vi "Start Stream.vi"(8 "error in (no error)":errorcluster, 10 "Camera Settings":T1={"Exposure Time (ms)"=100.0, "Binning"=enum."2x2", "Scan Mode"=0, "Frames to Acquire"=1000.0, "Pixel Correction"=FALSE, "Frames to Skip"=0, "File Path"=path "", "Duty cycle"=0.0, "ALEX"=FALSE, "Shutter Enable"=[], "fluidics trigger, ms (0=disabled)"=0.0, "Bit Depth"=0, "Image Width (px)"=0, "Image Height (px)"=0, "Horizontal Offset (px)"=0, "Vertical Offset (px)"=0} {"fluidics trigger, ms (0=disabled)" max=60000.0 step=1.0; "Exposure Time (ms)" min=1.0 max=10000.0 step=1.0}, 11 "Andor Camera in":refnum<class "Andor Camera.lvclass">) -> (0 "error out":errorcluster, 3 "Andor Camera out":refnum<class "Andor Camera.lvclass">)   [LabVIEW 2023, in "Andor Camera.lvlib" / "Andor Camera.lvclass"]
uses:
  Andor Camera.lvclass
  Resources/Type Defs/Camera Settings.ctl
  <userlib>/atmcd64d.llb/Spool_method typedef.ctl
  <userlib>/atmcd64d.llb/AcquisitionMode_mode typedef.ctl
  Camera/Camera.lvclass
  Andor Camera.lvclass/Andor Camera.ctl
panel:
  out "DLL error code 4":u32
  out "DLL error code 3":u32
  out "DLL error code 2":u32
  out "DLL error code":u32
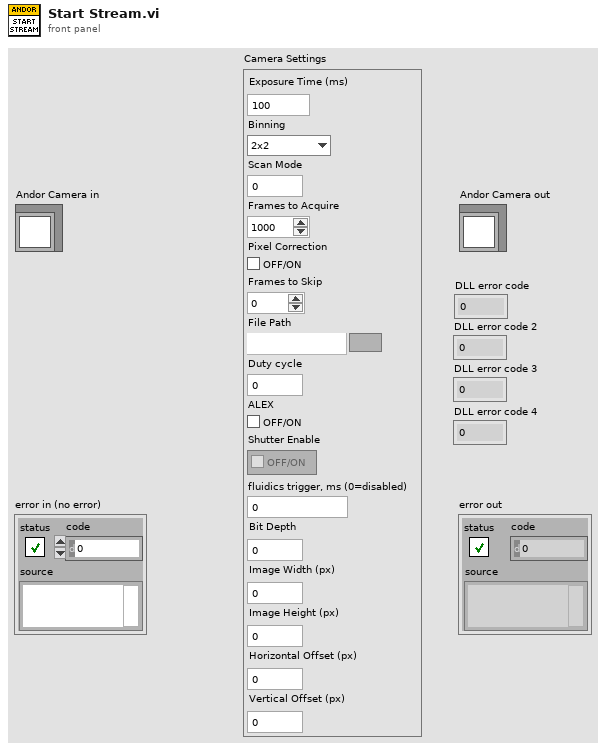
[diagram p1: front panel]
types:
  T1 = typedef "Camera Settings.ctl" = cluster{"Exposure Time (ms)":dbl, "Binning":enum16{"1x1", "2x2", "4x4"}, "Scan Mode":i32, "Frames to Acquire":dbl, "Pixel Correction":bool, "Frames to Skip":u32, "File Path":path, "Duty cycle":dbl, "ALEX":bool, "Shutter Enable":bool[], "fluidics trigger, ms (0=disabled)":dbl, "Bit Depth":u16, "Image Width (px)":u16, "Image Height (px)":u16, "Horizontal Offset (px)":u16, "Vertical Offset (px)":u16}
  T2 = typedef "AcquisitionMode_mode typedef.ctl" = enum16{"Reserved (0)", "Single Scan", "Accumulate", "Kinetics", "Fast Kinetics", "Run Till Abort", "Reserved (6)", "Reserved (7)", "Reserved (8)", "Time Delayed Integration"}
  T3 = typedef "Spool_method typedef.ctl" = enum16{"32-bit", "Depends", "16-bit", "Multiple Directory", "Spool to RAM disk", "16-bit FITS", "SIF", "16-buit TIFF", "Multiple Directory Compressed"}
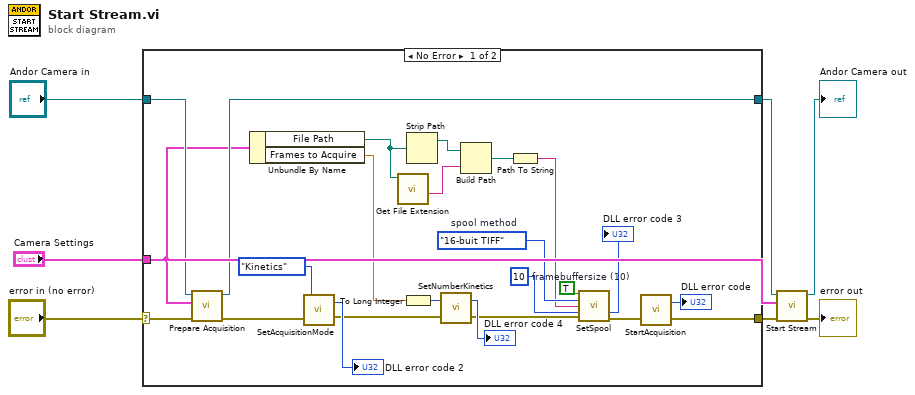
[diagram p0: block diagram]
diagram:
  n1 = case shown="No Error" "error in (no error)" {
    selector: "error in (no error)" -> [w31 w32]
    tunnel: "Camera Settings" -> [w27 _]
    tunnel: [w25 w32] -> w3
    tunnel: "Andor Camera in" -> [w29 w33]
    tunnel: [w28 w33] -> w1
    frame No Error {
      w23 = 10  # framebuffersize (10)
      w24 = Spool_method_typedef."16-buit TIFF"  # spool method
      n2 = call-dynamic "Prepare Acquisition.vi"("error in (no error)"=w31, "Camera Settings"=w27, "Andor Camera in"=w29) -> ("error out"=w30:errorcluster, "Andor Camera out"=w28:refnum<class "Andor Camera.lvclass">)  [unwired: 7 in]
      n3 = Unbundle By Name(w27) -> ("File Path"=w15:path, "Frames to Acquire"=w8:dbl)
      n4 = call <userlib>:"SetAcquisitionMode.vi"("error in (no error)"=w30, "mode"=AcquisitionMode_mode_typedef."Kinetics") -> ("error out"=w11:errorcluster, "DLL error code"=→"DLL error code 2":u32)
      n5 = call <vilib>:"Get File Extension.vi"("file"=w15) -> ("filename without extension"=w14:string)  [unwired: 6 in, 4 out]
      n6 = To Long Integer(number=w8) -> (32bit integer=w9:i32)
      n7 = Strip Path(path=w15) -> (stripped path=w16:path)  [unwired: 1 out]
      n8 = call <userlib>:"SetNumberKinetics.vi"("error in (no error)"=w11, "number"=w9) -> ("error out"=w10:errorcluster, "DLL error code"=→"DLL error code 4":u32)
      n9 = Build Path(base path=w16, name or relative path=w14) -> (appended path=w13:path)
      n10 = Path To String(path=w13) -> (string=w17:string)
      n11 = call <userlib>:"SetSpool.vi"("active"=TRUE, "method"=w24, "name"=w17, "framebuffersize (10)"=w23, "error in (no error)"=w10) -> ("DLL error code"=→"DLL error code 3":u32, "error out"=w26:errorcluster)  [unwired: 9 in]
      n12 = call <userlib>:"StartAcquisition.vi"("error in (no error)"=w26) -> ("error out"=w25:errorcluster, "DLL error code"=→"DLL error code":u32)  [unwired: 1 in]
    }
    frame Error {
    }
  }
  n13 = call-parent "Start Stream.vi"("error in (no error)"=w3, "Camera Settings"="Camera Settings", "Camera in"=w1) -> ("error out"=→"error out":errorcluster, "Camera out"=→"Andor Camera out":refnum<class "Andor Camera.lvclass">)  [unwired: 7 in]
